vi "dfd_Narrowband Filter Compute Delay.vi"(1 "multirate filters in":T1[](array[typedef]) {"mMRate_SumWl" min=1 max=32 step=1; "mMRate_InputIwl" min=1 max=32 step=1; "mMRate_GainWl" min=1 max=32 step=1; "mMRate_OutputWl" min=1 max=32 step=1; "mMRate_InputWl" min=1 max=32 step=1; "mMRate_CoefWl" min=1 max=32 step=1; "mMRate_Mode" items=["Default"=-1, "No Rate Change"=0, "Interpolation"=1, "Decimation"=2, "Interpolated"=3, "Rational"=4]}) -> (0 "#sample":i32)   [LabVIEW 2017, in "NI_DigFilter_Process.lvlib"]
uses:
  <vilib>/addons/Digital Filter Design/NI_DigFilter_Process.lvlib
  <vilib>/addons/Digital Filter Design/_Objects.llb/DFD Multirate Filter Obj.ctl
  <vilib>/addons/Digital Filter Design/_Objects.llb/DFD Multirate Mode.ctl
  <vilib>/addons/Digital Filter Design/_Objects.llb/DFD Coef Norm Type.ctl
  <vilib>/addons/Digital Filter Design/_Objects.llb/DFD Round-off Mode.ctl
  <vilib>/addons/Digital Filter Design/_Objects.llb/DFD FXP MRate Multiply Mode.ctl
  <vilib>/addons/Digital Filter Design/NI_DigFilterLicensed.lvlib
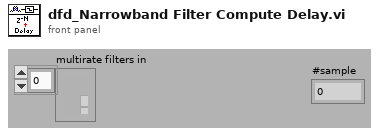
[diagram p1: front panel]
types:
  T1 = typedef "NI_DigFilterLicensed.lvlib/DFD Multirate Filter Obj.ctl" = cluster{"mMRate_Structure":enum16{"CIC", "FIR", "IIR", "Lattice"}, "mMRate_Mode":T2, "mMRate_Factor":i32, "mMRate_FIRParams":cluster{"mMRate_FIR_H":dbl[], "mMRate_FIR_IsNyquist?":bool, "mMRate_FIR_IsSymmetric?":bool}, "mMRate_CICParams":cluster{"mMRate_CIC_#Stage":i32, "mMRate_CIC_Lag":i32, "mMRate_CIC_Type":enum16{"Lowpass", "Highpass"}}, "mMRate_Order":i32, "mMRate_Version":string, "mMRate_Comments":string, "mMRate_RationalFactor":cluster{"mMRate_L":i32, "mMRate_M":i32}, "mMRate_Fs":dbl, "mMRate_Quantized?":bool, "mMRate_QFilterGain":dbl, "mMRate_CoefWl":i16, "mMRate_Scaling":cluster{"mMRate_ScaleByPowerOf2?":bool, "mMRate_ScaleType":T3}, "mMRate_InputWl":i16, "mMRate_OutputWl":i16, "mMRate_OutputMode":T4, "mMRate_MultMode":T5, "mMRate_BitPruning":bool, "mMRate_GainWl":i16, "mMRate_OutputFwl":i16, "mMRate_SumIwl":i16, "mMRate_InputIwl ":i16, "mMRate_SumWl":i16, "mMRate_CoefIwl":i16}
  T2 = typedef "NI_DigFilterLicensed.lvlib/DFD Multirate Mode.ctl" = i16
  T3 = typedef "NI_DigFilterLicensed.lvlib/DFD Coef Norm Type.ctl" = enum16{"No Norm", "Time Domain 1-Norm", "Time Domain 2-Norm", "Time Domain Inf-Norm"}
  T4 = typedef "NI_DigFilterLicensed.lvlib/DFD Round-off Mode.ctl" = enum16{"Nearest", "Truncation"}
  T5 = typedef "NI_DigFilterLicensed.lvlib/DFD FXP MRate Multiply Mode.ctl" = enum16{"Truncated", "Full"}
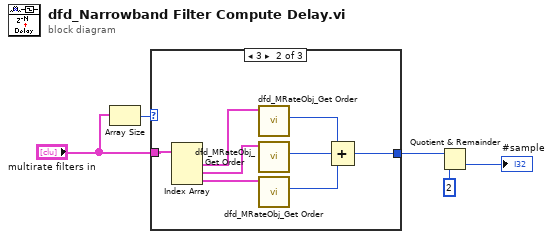
[diagram p0: block diagram]
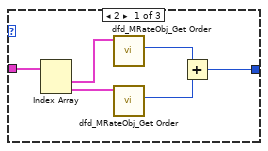
[diagram p2: hidden frame]
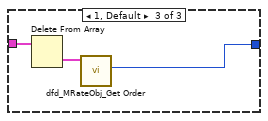
[diagram p3: hidden frame]
diagram:
  n1 = Array Size(array="multirate filters in") -> (size(s)=w4:i32)
  n2 = case shown="3" w4 {
    tunnel: "multirate filters in" -> [w11 w19 w22]
    tunnel: [w8 w15 w20] -> w2
    frame 2 {
      n3 = Index Array(array=w11) -> (element #1=w9:T1, element #2=w10:T1)  [unwired: 2 in]
      n4 = call <vilib>:"dfd_MRateObj_Get Order.vi"("multirate filter in"=w9) -> ("order"=w6:i32)  [unwired: 10 out]
      n5 = call <vilib>:"dfd_MRateObj_Get Order.vi"("multirate filter in"=w10) -> ("order"=w7:i32)  [unwired: 10 out]
      n6 = Add(x=w6, y=w7) -> (x+y=w8:i32)
    }
    frame 3 {
      n7 = Index Array(array=w19) -> (element #1=w18:T1, element #2=w17:T1, element #3=w16:T1)  [unwired: 3 in]
      n8 = call <vilib>:"dfd_MRateObj_Get Order.vi"("multirate filter in"=w18) -> ("order"=w14:i32)  [unwired: 10 out]
      n9 = call <vilib>:"dfd_MRateObj_Get Order.vi"("multirate filter in"=w17) -> ("order"=w13:i32)  [unwired: 10 out]
      n10 = call <vilib>:"dfd_MRateObj_Get Order.vi"("multirate filter in"=w16) -> ("order"=w12:i32)  [unwired: 10 out]
      n11 = Compound Arithmetic op=ADD(w14, w13, w12) -> (w15:i32)
    }
    frame 1, Default {
      n12 = Delete From Array(array=w22) -> (deleted portion=w21:T1)  [unwired: 2 in, 1 out]
      n13 = call <vilib>:"dfd_MRateObj_Get Order.vi"("multirate filter in"=w21) -> ("order"=w20:i32)  [unwired: 10 out]
    }
  }
  n14 = Quotient & Remainder(x=w2, y=2) -> (floor(x/y)=→"#sample":i32)  [unwired: 1 out]
